vi "Example.vi"() -> ()   [LabVIEW 2018]
uses:
  Data Def/EPS-Value Type.ctl
  Data Def/EPS-Setting.ctl
panel:
  out "Stop":bool
  out "Setting":T1
  in  "Apply":bool
  out "Input?":bool
  in  "Stop Load":bool
  in  "Apply Load":bool
  out "Data":T1(graph)
  out "Value Type State":T2
  in  "Values":dbl format="%#.3g"
  in  "Operation Mode":T2
  out "Mode":string
  out "Device Information":T3
  in  "Port":u16=5025
  in  "IP Address":string="192.168.3.249"
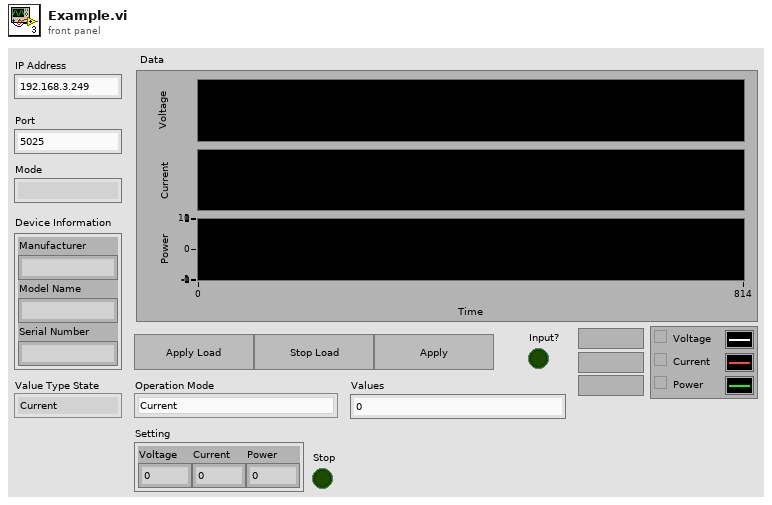
[diagram p1: front panel]
types:
  T1 = cluster{"Voltage":dbl, "Current":dbl, "Power":dbl}
  T2 = typedef "EPS-Value Type.ctl" = enum16{"Current", "Vlotage", "Power"}
  T3 = cluster{"Manufacturer":string, "Model Name":string, "Serial Number":string}
  T4 = typedef "EPS-Setting.ctl" = cluster{"IP Address":string, "Port":u16, "Connection ID":refnum<k5>}
  T5 = typedef "EPS-Measurement Data.ctl" = cluster{"Voltage":dbl, "Current":dbl, "Power":dbl}
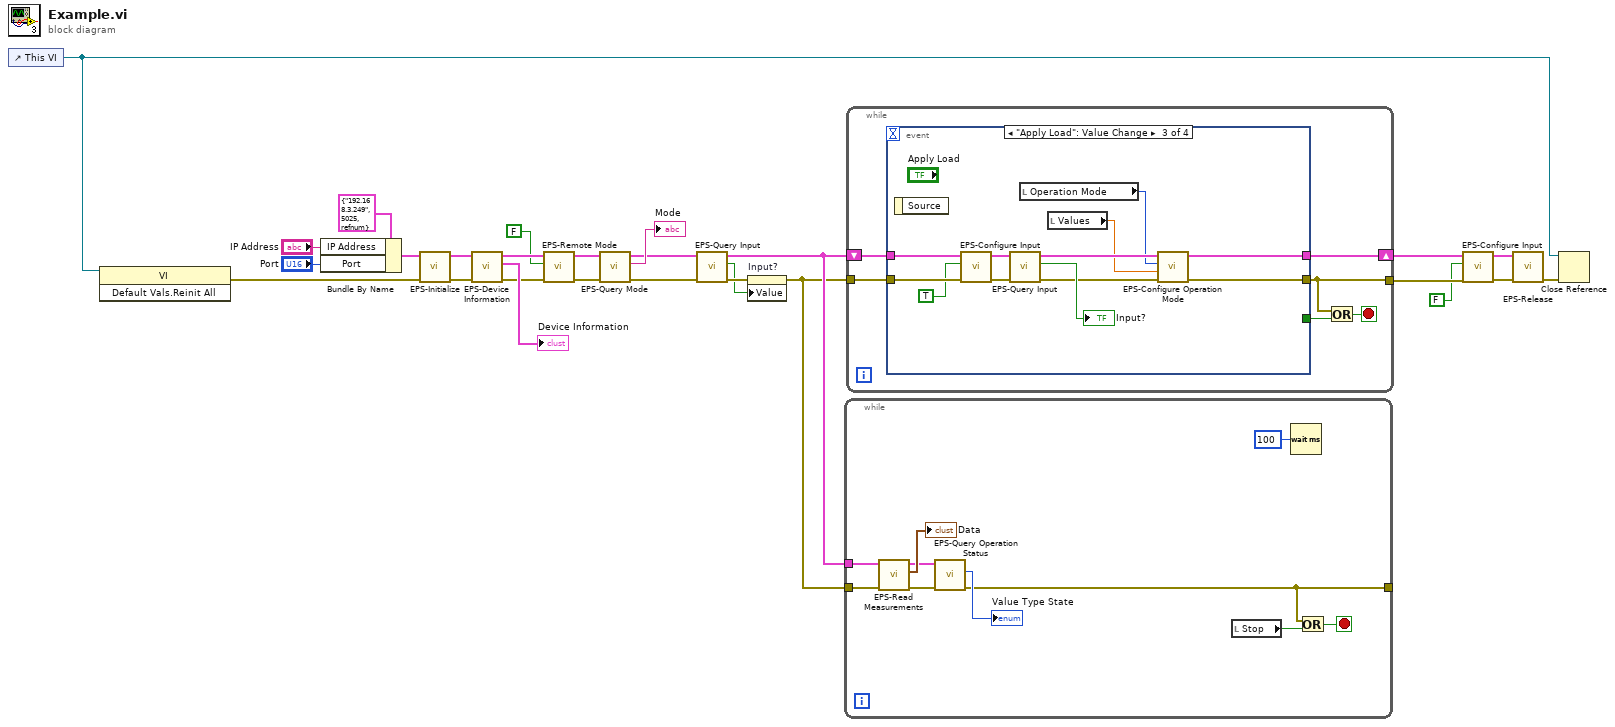
[diagram p0: block diagram]
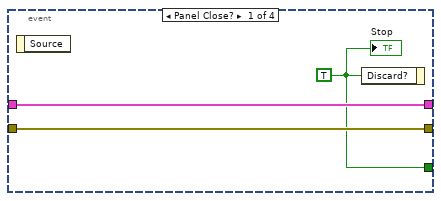
[diagram p2: hidden frame]
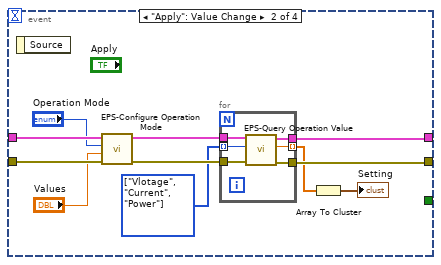
[diagram p3: hidden frame]
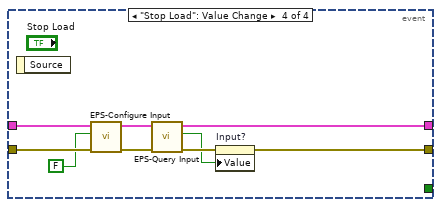
[diagram p4: hidden frame]
diagram:
  n1 = control-ref of="This VI"() -> (w12:refnum<vi>)
  n2 = invoke class="VI" method="Default Vals.Reinit All"(reference=w12) -> (error out=w14:errorcluster)  [unwired: 2 in, 2 out]
  n3 = Bundle By Name(cluster=T4 {"IP Address"="192.168.3.249", "Port"=5025, "Connection ID"=refnum} ("EPS Setting In"), "IP Address"="IP Address", "Port"="Port") -> (w24:T4)
  n4 = call "EPS-Initialize.vi"("error in"=w14, "EPS Setting In"=w24) -> ("error out"=w26:errorcluster, "EPS Setting Out"=w27:T4)  [unwired: 8 in]
  n5 = call "EPS-Device Information.vi"("error in"=w26, "EPS Setting In"=w27) -> ("error out"=w19:errorcluster, "Device Information"=→"Device Information":T3, "EPS Setting Out"=w20:T4)  [unwired: 7 in]
  n6 = call "EPS-Remote Mode.vi"("error in"=w19, "Remote"=FALSE, "EPS Setting In"=w20) -> ("error out"=w16:errorcluster, "EPS Setting Out"=w17:T4)  [unwired: 7 in]
  n7 = call "EPS-Query Mode.vi"("error in"=w16, "EPS Setting In"=w17) -> ("error out"=w5:errorcluster, "Mode"=→"Mode":string, "EPS Setting Out"=w6:T4)  [unwired: 7 in]
  n8 = call "EPS-Query Input.vi"("error in"=w5, "EPS Setting In"=w6) -> ("error out"=w4:errorcluster, "Input?"=w3:bool, "EPS Setting Out"=w2:T4)  [unwired: 7 in]
  n9 = property on="Input?" class="Bool (strict)"(error in=w4, "Value"=w3) -> (error out=w1:errorcluster)  [unwired: 1 in, 1 out]
  n10 = while {
    tunnel: w2 -> [w33]
    tunnel: w1 -> [w32]
    tunnel: [w31] -> _
    stop <- w29 stop-if-true
    n11 = call "EPS-Read Measurements.vi"("error in"=w32, "EPS Setting In"=w33) -> ("error out"=w35:errorcluster, "Measurement Data"=→"Data":T5, "EPS Setting Out"=w34:T4)  [unwired: 7 in]
    n12 = call "EPS-Query Operation Status.vi"("error in"=w35, "EPS Setting In"=w34) -> ("error out"=w31:errorcluster, "Value Type"=→"Value Type State":T2)  [unwired: 6 in, 2 out]
    n13 = local read "Stop"() -> (w30:bool)
    n14 = Wait (ms)(milliseconds to wait=u32 100) -> ()  [unwired: 1 out]
    n15 = Or(x=w31, y=w30) -> (x .or. y?=w29:bool)
  }
  n16 = while {
    shift-right: [w41] -> w11
    shift-left: w2 -> [w43]
    tunnel: w1 -> [w42]
    tunnel: [w40] -> w10
    stop <- w38 stop-if-true
    n17 = event shown="[2] \"Apply Load\": Value Change" {
      selector: _ -> [_ _ _ _]
      dyn-events: _ -> [_ _ _ _]
      timeout: _ -> [_ _ _ _]
      tunnel: w43 -> [w45 w57 w74 w83]
      tunnel: w42 -> [w46 w56 w75 w84]
      tunnel: [w46 w50 w67 w76] -> w40
      tunnel: [w45 w51 w66 w77] -> w41
      tunnel: [w44 _ _ _] -> w39
      event Panel Close? {
        w44 = TRUE ("Discard?")
        n18 = event-data() -> ()  [unwired: 1 in, 1 out]
        n19 = event-data("Discard?"=w44) -> ()  [unwired: 1 in, 1 out]
        "Stop" <- w44
      }
      event "Apply": Value Change {
        w49 = T2[] [enum."Vlotage", enum."Current", enum."Power"] items=["Current", "Vlotage", "Power"] ("Array")
        n20 = event-data() -> ()  [unwired: 1 in, 1 out]
        n21 = call "EPS-Configure Operation Mode.vi"("error in"=w56, "Values"="Values", "Operation Mode"="Operation Mode", "EPS Setting In"=w57) -> ("error out"=w52:errorcluster, "EPS Setting Out"=w53:T4)  [unwired: 6 in]
        n22 = for {
          tunnel: w53 -> [w62]
          tunnel: w52 -> [w63]
          tunnel: [w61] -> w51
          tunnel: [w60] -> w50
          tunnel: w49 -> [w59] mode=indexing
          tunnel: [w58] -> w48 mode=indexing
          n23 = call "EPS-Query Operation Value.vi"("error in"=w63, "Value Type"=w59, "EPS Setting In"=w62) -> ("error out"=w60:errorcluster, "Value"=w58:dbl, "EPS Setting Out"=w61:T4)  [unwired: 6 in]
        }
        n24 = Array To Cluster(array=w48) -> (cluster=→"Setting":cluster{"[0]":dbl, "[1]":dbl, "[2]":dbl})
      }
      event "Apply Load": Value Change {
        n25 = event-data() -> ()  [unwired: 1 in, 1 out]
        n26 = call "EPS-Configure Input.vi"("error in"=w75, "Enable Input"=TRUE, "EPS Setting In"=w74) -> ("error out"=w71:errorcluster, "EPS Setting Out"=w72:T4)  [unwired: 7 in]
        n27 = call "EPS-Query Input.vi"("error in"=w71, "EPS Setting In"=w72) -> ("error out"=w68:errorcluster, "Input?"=→"Input?":bool, "EPS Setting Out"=w69:T4)  [unwired: 7 in]
        n28 = local read "Operation Mode"() -> (w64:T2)
        n29 = local read "Values"() -> (w65:dbl)
        n30 = call "EPS-Configure Operation Mode.vi"("error in"=w68, "Values"=w65, "Operation Mode"=w64, "EPS Setting In"=w69) -> ("error out"=w67:errorcluster, "EPS Setting Out"=w66:T4)  [unwired: 6 in]
      }
      event "Stop Load": Value Change {
        n31 = event-data() -> ()  [unwired: 1 in, 1 out]
        n32 = call "EPS-Configure Input.vi"("error in"=w84, "Enable Input"=FALSE, "EPS Setting In"=w83) -> ("error out"=w80:errorcluster, "EPS Setting Out"=w81:T4)  [unwired: 7 in]
        n33 = call "EPS-Query Input.vi"("error in"=w80, "EPS Setting In"=w81) -> ("error out"=w79:errorcluster, "Input?"=w78:bool, "EPS Setting Out"=w77:T4)  [unwired: 7 in]
        n34 = property on="Input?" class="Bool (strict)"(error in=w79, "Value"=w78) -> (error out=w76:errorcluster)  [unwired: 1 in, 1 out]
      }
    }
    n35 = Or(x=w40, y=w39) -> (x .or. y?=w38:bool)
  }
  n36 = call "EPS-Configure Input.vi"("error in"=w10, "Enable Input"=FALSE, "EPS Setting In"=w11) -> ("error out"=w9:errorcluster, "EPS Setting Out"=w8:T4)  [unwired: 7 in]
  n37 = call "EPS-Release.vi"("error in"=w9, "EPS Setting"=w8) -> ("error out"=w13:errorcluster)  [unwired: 9 in]
  n38 = Close Reference(reference=w12, error in (no error)=w13) -> ()  [unwired: 1 out]
